vi "Filter.vi"(8 "滤波":bool, 11 "ID(Hex 高位有效)":string="40A") -> (0 "屏蔽码":u32 format="%.0x", 3 "验收码":u32 format="%.0x")   [LabVIEW 2013]
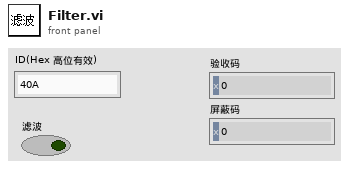
[diagram p1: front panel]
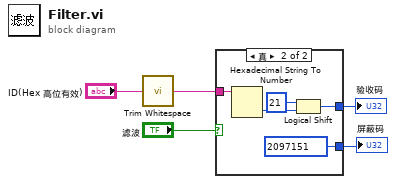
[diagram p0: block diagram]
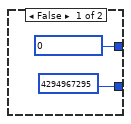
[diagram p2: hidden frame]
diagram:
  n1 = call <vilib>:"Trim Whitespace.vi"("string"="ID(Hex 高位有效)") -> ("trimmed string"=w4:string)  [unwired: 1 in]
  n2 = case shown="真" "滤波" {
    tunnel: w4 -> [_ w10]
    tunnel: [u32 0 ("验收码") w9] -> w2
    tunnel: [u32 4294967295 ("屏蔽码") u32 2097151 ("屏蔽码")] -> w1
    frame False {
    }
    frame True {
      n3 = Hexadecimal String To Number(string=w10) -> (number=w12:u32)  [unwired: 2 in, 1 out]
      n4 = Logical Shift(y=i8 21, x=w12) -> (x << y=w9:u32)
    }
  }
  "验收码" <- w2
  "屏蔽码" <- w1
